vi "dummy_handle_pose.vi"(1 "Initial output pose":T1) -> (0 "Dummy handle pose":T1)   [LabVIEW 2013]
uses:
  <vilib>/Analysis/Matrix/Datatypes/RealMatrix.ctl
  <vilib>/Analysis/Matrix/NI_Matrix.lvlib
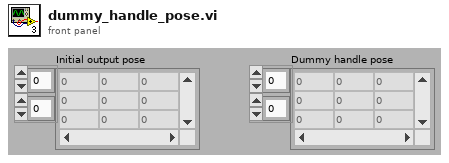
[diagram p1: front panel]
types:
  T1 = typedef "NI_Matrix.lvlib/RealMatrix.ctl" = dbl[][]
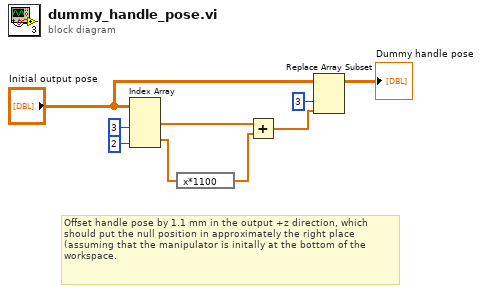
[diagram p0: block diagram]
diagram:
  # "Offset handle pose by 1.1 mm in the output +z direction, which should put the null position in approximately the right place (assuming that the manipulator is initally at the bottom of the workspace."
  n1 = Index Array(array="Initial output pose", index (col) #1=3 ("disabled index (col)"), index (col) #2=2 ("index (col)")) -> (element #1=w6:dbl[], element #2=w7:dbl[])  [unwired: 2 in]
  n2 = expression code="x*1100"(w7) -> (w5:dbl[])
  n3 = Add(x=w6, y=w5) -> (x+y=w2:dbl[])
  n4 = Replace Array Subset(array="Initial output pose", new element=w2, index (col)=3 ("disabled index (col)")) -> (→"Dummy handle pose":T1)  [unwired: 1 in]
